vi "Generate User Event.vi"(8 "error in (no error)":errorcluster, 10 "Data":variant, 11 "Message":T1) -> (0 "error out":errorcluster)   [LabVIEW 2010, in "Error Handler.lvlib"]
uses:
  Error Handler.lvlib
  Event Ref FGV Command Enum.ctl
  User Event Message Enum.ctl
  User Event Message Cluster.ctl
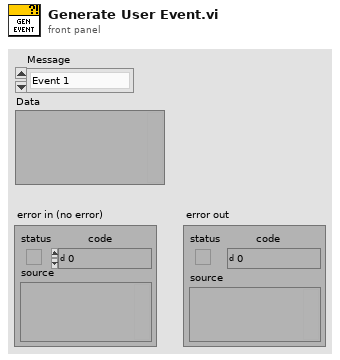
[diagram p1: front panel]
types:
  T1 = typedef "Error Handler.lvlib/User Event Message Enum.ctl" = enum16{"Event 1"}
  T2 = typedef "Error Handler.lvlib/User Event Message Cluster.ctl" = cluster{"Enum":T1, "Data":variant}
  T3 = typedef "Error Handler.lvlib/Event Ref FGV Command Enum.ctl" = enum16{"Create Event", "Get Event Ref", "Release Event"}
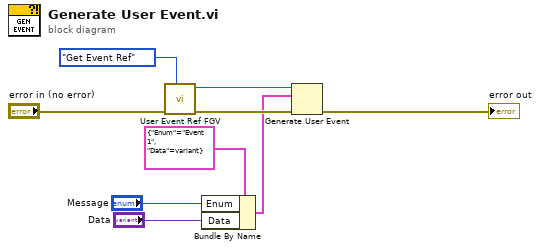
[diagram p0: block diagram]
diagram:
  n1 = call "User Event Ref FGV.vi"("Command"=Event_Ref_FGV_Command_Enum."Get Event Ref", "error in (no error)"="error in (no error)") -> ("error out"=w6:errorcluster, "User Event"=w7:refnum<user-event>)  [unwired: 8 in]
  n2 = Bundle By Name(cluster=T2 {"Enum"=enum."Event 1", "Data"=variant} ("event data"), "Enum"="Message", "Data"="Data") -> (w2:T2)
  n3 = Generate User Event(user event=w7, event data cluster=w2, error in=w6) -> (error out=→"error out":errorcluster)  [unwired: 1 out]
